vi "_VISA Write.vi"(8 "error in (no error)":errorcluster, 10 "write buffer":string, 11 "VISA resource name":refnum<visa-resource-name>="GPIB0::23::INSTR") -> (0 "error out":errorcluster, 2 "return count":u32, 3 "VISA resource name out":refnum<visa-resource-name>)   [LabVIEW 2017, in "SR400.lvlib"]
uses:
  SR400.lvlib
  Global/GPIB Numbers.vi
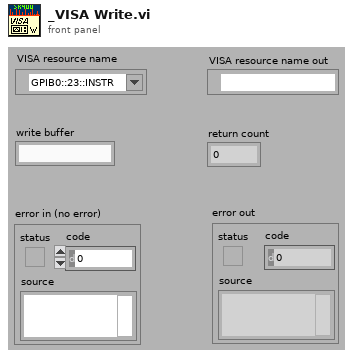
[diagram p1: front panel]
types:
  T1 = typedef "GPIB Type Def.ctl" = cluster{"Name":string, "bus":dbl, "GPIB":dbl, "GPIB as string":string, "byte":i32, "VISA Resource Name":refnum<visa-resource-name>}
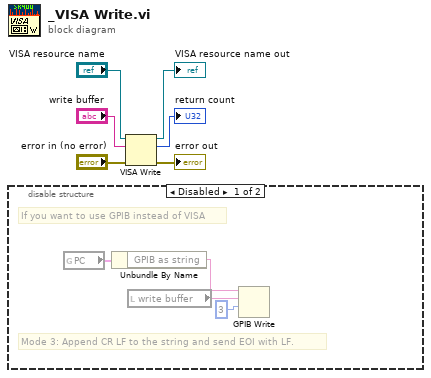
[diagram p0: block diagram]
diagram:
  n1 = disable-structure shown="Disabled" {
    frame Disabled {
      # "Mode 3: Append CR LF to the string and send EOI with LF."
      # "If you want to use GPIB instead of VISA"
      n2 = global read "GPIB Numbers.vi" "PC"() -> (w10:T1)
      n3 = Unbundle By Name(w10) -> ("GPIB as string"=w9:string)
      n4 = local read "write buffer"() -> (w8:string)
      n5 = GPIB Write(0:w9, 1:w8, 2:i16 3 ("mode (0)")) -> ()  [unwired: 1 in, 3 out]
    }
    frame Enabled {
    }
  }
  n6 = VISA Write(VISA resource name="VISA resource name", write buffer="write buffer", error in (no error)="error in (no error)") -> (VISA resource name out=→"VISA resource name out":refnum<visa-resource-name>, return count=→"return count":u32, error out=→"error out":errorcluster)
